vi "Pretty Print JSON.vi"(8 "error in (no error)":errorcluster, 10 "JSON in":string, 11 "String in":refnum<vi>) -> (0 "error out":errorcluster)   [LabVIEW 2018]
uses:
  <vilib>/JDP Science/JSONtext/JSONtext.lvlib
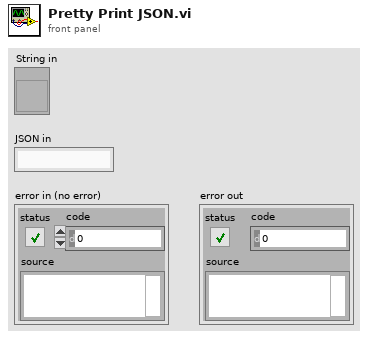
[diagram p1: front panel]
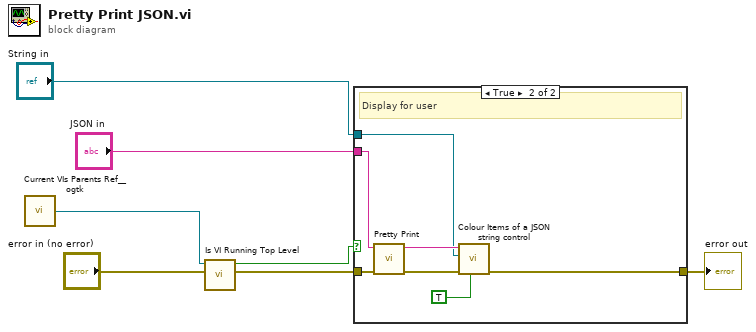
[diagram p0: block diagram]
diagram:
  n1 = call <userlib>:"Current VIs Parents Ref__ogtk.vi"() -> ("Calling VI's Reference"=w1:refnum<vi>)  [unwired: 2 in]
  n2 = call "Is VI Running Top Level.vi"("Error in"="error in (no error)", "VI to Check"=w1) -> ("Error out"=w2:errorcluster, "Top Level"=w4:bool)  [unwired: 8 in]
  n3 = case shown="True" w4 {
    tunnel: "JSON in" -> [_ w15]
    tunnel: w2 -> [w8 w12]
    tunnel: [w8 w10] -> w5
    tunnel: "String in" -> [_ w9]
    frame False {
    }
    frame True {
      # "Display for user"
      n4 = call <vilib>:"Pretty Print.vi"("error in (no error)"=w12, "JSON"=w15) -> ("error out"=w11:errorcluster, "<JSON>"=w14:string)  [unwired: 7 in, 1 out]
      n5 = call <vilib>:"Colour Items of a JSON string control.vi"("Defer Panel Updates"=TRUE, "error in (no error)"=w11, "String Control"=w9, "JSON"=w14) -> ("error out"=w10:errorcluster)  [unwired: 7 in]
    }
  }
  "error out" <- w5
